vi "_ RunMe.vi"() -> ()   [LabVIEW 2016]
uses:
  USER32.DLL
panel:
  out "hWnd 3":u32
  out "error out":errorcluster
  out "hWnd 2":u32
  out "hWnd":u32
  in  "Image":path=path "C:/Users/Marco Preziani/Documents/VLC Snapshots/butta.jpg"
  in  "Dest Format":string(combo)="{6fddc324-4e03-4bfe-b185-3d77768dc90e}"
  out "Image":T1(plugin-control)
  out "Image Stride":u32
  out "Image Height":u32
  out "Image Width":u32
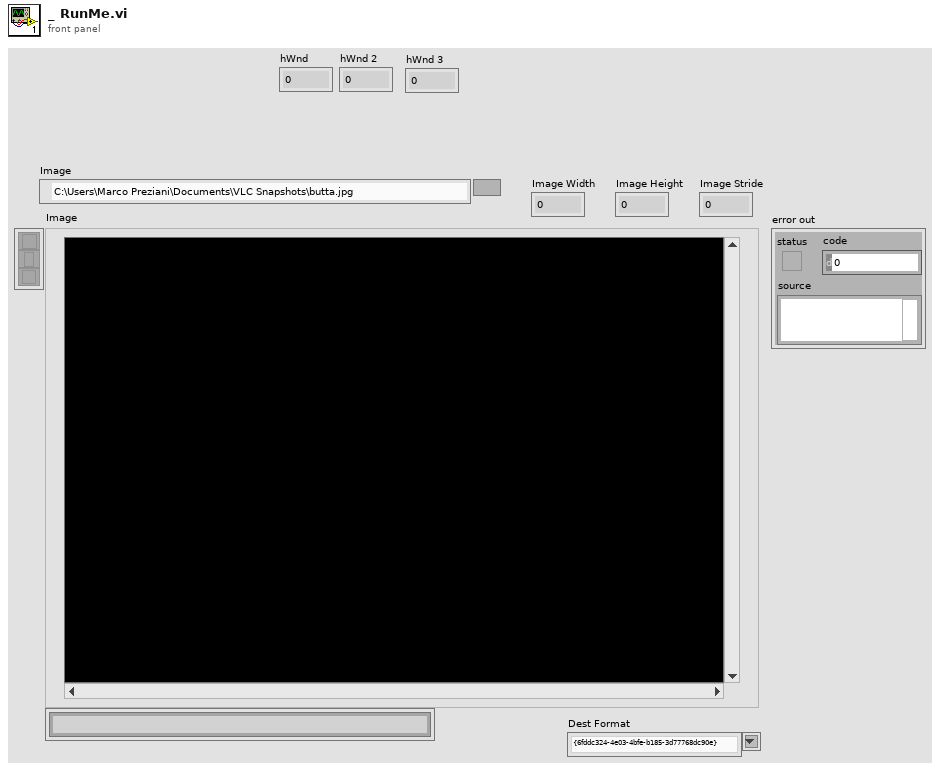
[diagram p1: front panel]
types:
  T1 = typedef "IMAQ Image.ctl" = refnum<image>
  T2 = typedef "Image Type" = u32
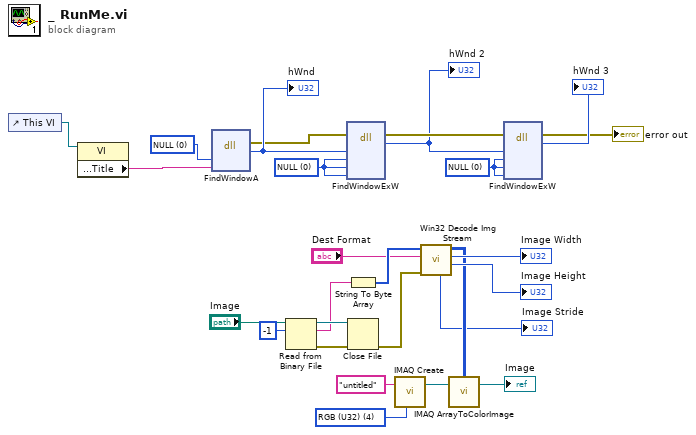
[diagram p0: block diagram]
diagram:
  w4 = 0 items=["NULL"]
  w8 = 0 items=["NULL"]
  w11 = 0 items=["NULL"]
  w19 = T2 4 items=["Grayscale (U8)", "Grayscale (I16)", "Grayscale (SGL)", "Complex (CSG)", "RGB (U32)", "HSL (U32)", "RGB (U64)", "Grayscale (U16)"] ("Image Type")
  n1 = control-ref of="This VI"() -> (w3:refnum<vi>)
  n2 = property class="VI"(reference=w3) -> ("Front Panel Window:Title"=w10:string)  [unwired: 1 in, 2 out]
  n3 = dll-call lib="USER32.DLL" fn="FindWindowA" label="FindWindow"("lpszClassName"=w11, "lpszWindowName"=w10) -> (error out=w7:errorcluster, "hWnd"=w9:u32)  [unwired: 5 in, 1 out]
  "hWnd" <- w9
  n4 = Read from Binary File(10:-1 ("count (1)"), 11:"Image") -> (0:w13:errorcluster, 2:w24:string, 3:w25:refnum<file>)  [unwired: 4 in, 1 out]
  n5 = dll-call lib="user32.dll" fn="FindWindowExW" label="FindWindowEx"(error in=w7, "hwndParent"=w9, "hwndChildAfter"=w8, "lpszClassName"=w8, "lpszWindowName"=w8) -> (error out=w6:errorcluster, "hWnd"=w5:u32)  [unwired: 6 in, 1 out]
  "hWnd 2" <- w5
  n6 = String To Byte Array(string=w24) -> (unsigned byte array=w23:u8[])
  n7 = Close File(refnum=w25, error in=w13) -> (error out=w12:errorcluster)  [unwired: 1 out]
  n8 = call "IMAQ Create"("Image Name"="untitled", "Image Type"=w19) -> ("New Image"=w18:T1)  [unwired: 3 in, 1 out]
  n9 = call "Win32 Decode Img Stream.vi"("error in (no error)"=w12, "Dest Format"="Dest Format", "Image Data"=w23) -> ("Image Height"=→"Image Height":u32, "Image Width"=→"Image Width":u32, "Dest"=w16:u32[][], "Image Stride"=→"Image Stride":u32)  [unwired: 4 in, 1 out]
  n10 = call "IMAQ ArrayToColorImage"("Image Pixels (U32)"=w16, "Image"=w18) -> ("Image Out"=→"Image":T1)  [unwired: 3 in, 1 out]
  n11 = dll-call lib="user32.dll" fn="FindWindowExW" label="FindWindowEx"(error in=w6, "hwndParent"=w5, "hwndChildAfter"=w4, "lpszClassName"=w4, "lpszWindowName"=w4) -> (error out=→"error out":errorcluster, "hWnd"=→"hWnd 3":u32)  [unwired: 6 in, 1 out]
